vi "SetValue.vi"(0 "class data in":refnum<class "AnalogComparator.lvclass">, 5 "Value":dbl, 11 "error in (no error)":errorcluster) -> (4 "class data out":refnum<class "AnalogComparator.lvclass">, 15 "error out":errorcluster)   [LabVIEW 2019, in "AnalogComparator.lvclass"]
uses:
  AnalogComparator.lvclass
  AnalogComparator.lvclass/AnalogComparator.ctl
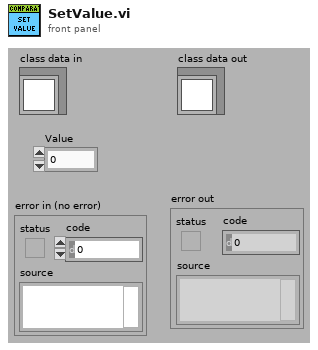
[diagram p1: front panel]
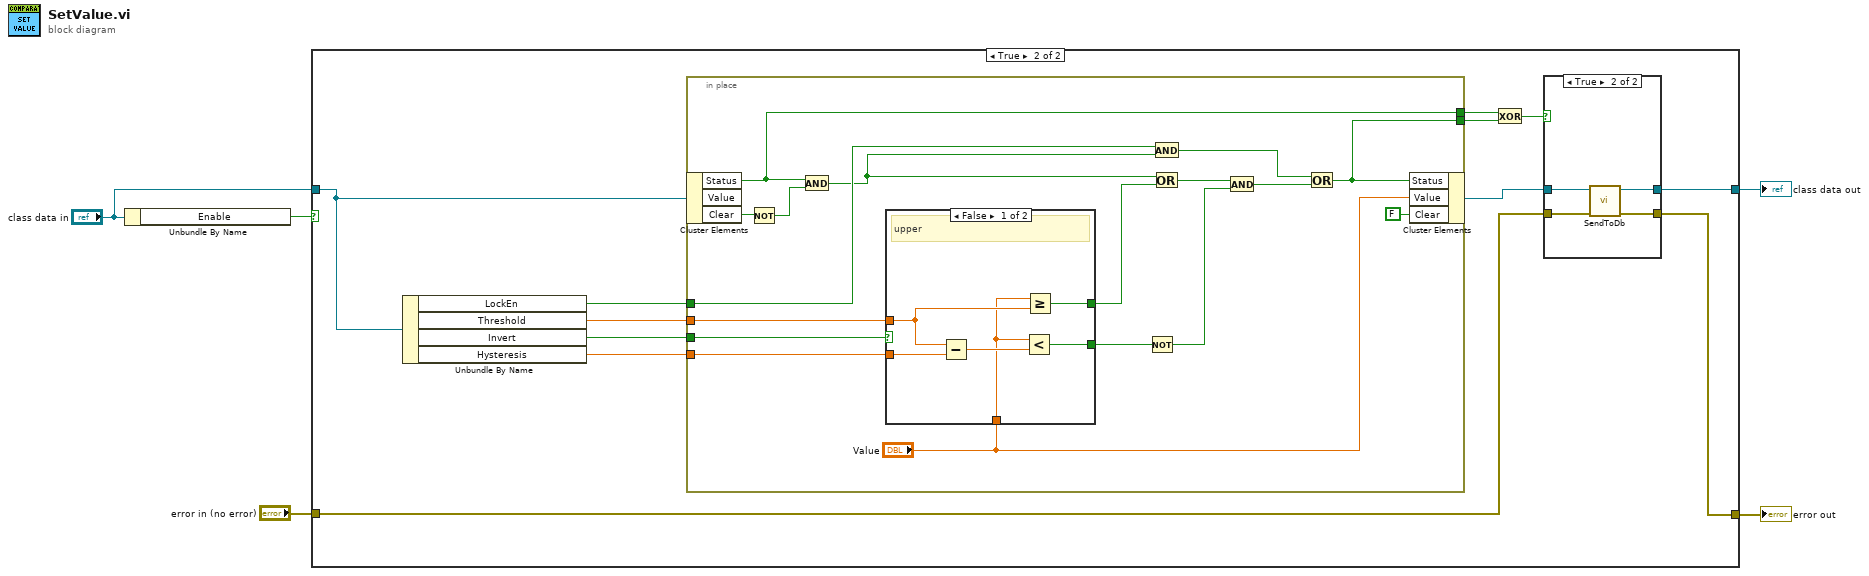
[diagram p0: block diagram]
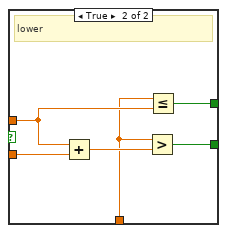
[diagram p4: hidden frame]
diagram:
  n1 = Unbundle By Name("class data in") -> ("Enable"=w4:bool)
  n2 = case shown="True" w4 {
    tunnel: [w7 w13] -> w5
    tunnel: "class data in" -> [w7 w19]
    tunnel: "error in (no error)" -> [w6 w12]
    tunnel: [w6 w11] -> w1
    frame False {
    }
    frame True {
      n3 = Unbundle By Name(w19) -> ("LockEn"=w15:bool, "Threshold"=w17:dbl, "Invert"=w16:bool, "Hysteresis"=w18:dbl)
      n4 = in-place {
        in-place-border: w17 -> [w42]
        in-place-border: w18 -> [w41]
        in-place-border: w16 -> [w35]
        in-place-border: w15 -> [w33]
        in-place-border: [w31] -> w10
        in-place-border: [w30] -> w9
        n5 = in-place-cluster #1(w19) -> ("Status"=w30:bool, "Clear"=w26:bool)  [unwired: 1 out]
        n6 = Not(x=w26) -> (.not. x?=w28:bool)
        n7 = And(x=w30, y=w28) -> (x .and. y?=w29:bool)
        n8 = case shown="False" w35 {
          tunnel: "Value" -> [w44 w50]
          tunnel: w42 -> [w45 w51]
          tunnel: w41 -> [w48 w54]
          tunnel: [w46 w52] -> w39
          tunnel: [w43 w49] -> w34
          frame False {
            # "upper"
            n9 = Subtract(x=w45, y=w48) -> (x-y=w47:dbl)
            n10 = Less?(x=w44, y=w47) -> (x < y?=w46:bool)
            n11 = Greater Or Equal?(x=w44, y=w45) -> (x >= y?=w43:bool)
          }
          frame True {
            # "lower"
            n12 = Add(x=w51, y=w54) -> (x+y=w53:dbl)
            n13 = Greater?(x=w50, y=w53) -> (0:w52:bool)
            n14 = Less Or Equal?(x=w50, y=w51) -> (x <= y?=w49:bool)
          }
        }
        n15 = Not(x=w39) -> (.not. x?=w38:bool)
        n16 = And(x=w33, y=w29) -> (x .and. y?=w36:bool)
        n17 = Or(x=w29, y=w34) -> (x .or. y?=w40:bool)
        n18 = And(x=w40, y=w38) -> (x .and. y?=w37:bool)
        n19 = Or(x=w36, y=w37) -> (x .or. y?=w31:bool)
        n20 = in-place-cluster #1("Status"=w31, "Value"="Value", "Clear"=FALSE) -> (w14:refnum<class "AnalogComparator.lvclass">)
      }
      n21 = Exclusive Or(1:w10, 2:w9) -> (0:w8:bool)
      n22 = case shown="True" w8 {
        tunnel: w14 -> [w21 w25]
        tunnel: [w21 w24] -> w13
        tunnel: w12 -> [w20 w23]
        tunnel: [w20 w22] -> w11
        frame False {
        }
        frame True {
          n23 = call "SendToDb.vi"("error in (no error)"=w23, "AnalogComparator in"=w25) -> ("error out"=w22:errorcluster, "AnalogComparator out"=w24:refnum<class "AnalogComparator.lvclass">)  [unwired: 8 in]
        }
      }
    }
  }
  "class data out" <- w5
  "error out" <- w1
